vi "Notify Observers (Root).vi"(7 "Type":enum16{"Event", "State"}(ring)=enum."State", 8 "error in (no error)":errorcluster, 10 "Array of State Messages":refnum<class "MSG.lvclass">[](array[class]), 11 "ObserverRegistry in":refnum<class "ObserverRegistry.lvclass">) -> (0 "error out":errorcluster, 3 "ObserverRegistry out":refnum<class "ObserverRegistry.lvclass">)   [LabVIEW 2011, in "Messenging.lvlib" / "ObserverRegistry.lvclass"]
uses:
  ObserverRegistry.lvclass
  Registration Entry.ctl
  Interprocess Messenger/TextVarientMessage/MSG.lvclass
  Interprocess Messenger/SendOnly/Observer.lvclass
  Interprocess Messenger/ErrorMessage/ErrorMessage.lvclass
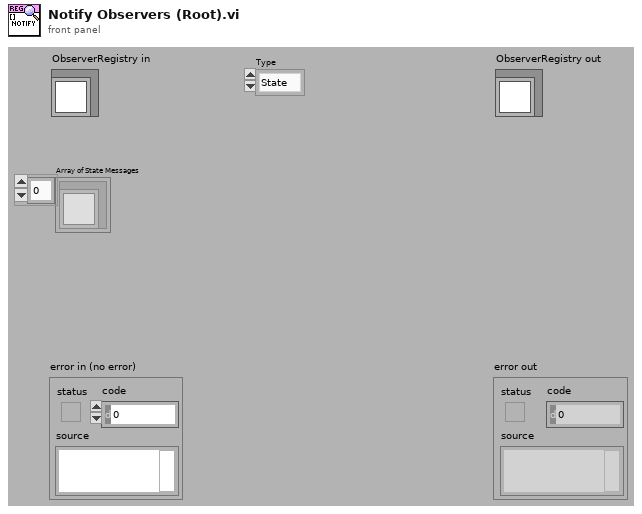
[diagram p1: front panel]
types:
  T1 = typedef "Messenging.lvlib/ObserverRegistry.lvclass/Registration Entry.ctl" = cluster{"Observer":refnum<class "Observer.lvclass">, "Type":enum16{"Event", "State"}, "Latest (State)":refnum<class "MSG.lvclass">}
  T2 = typedef "Messenging.lvlib/ObserverRegistry.lvclass/ObserverRegistryData.ctl" = cluster{"Observer of Errors":refnum<class "Observer.lvclass">, "Observer of All":refnum<class "Observer.lvclass">, "Event Registry":variant}
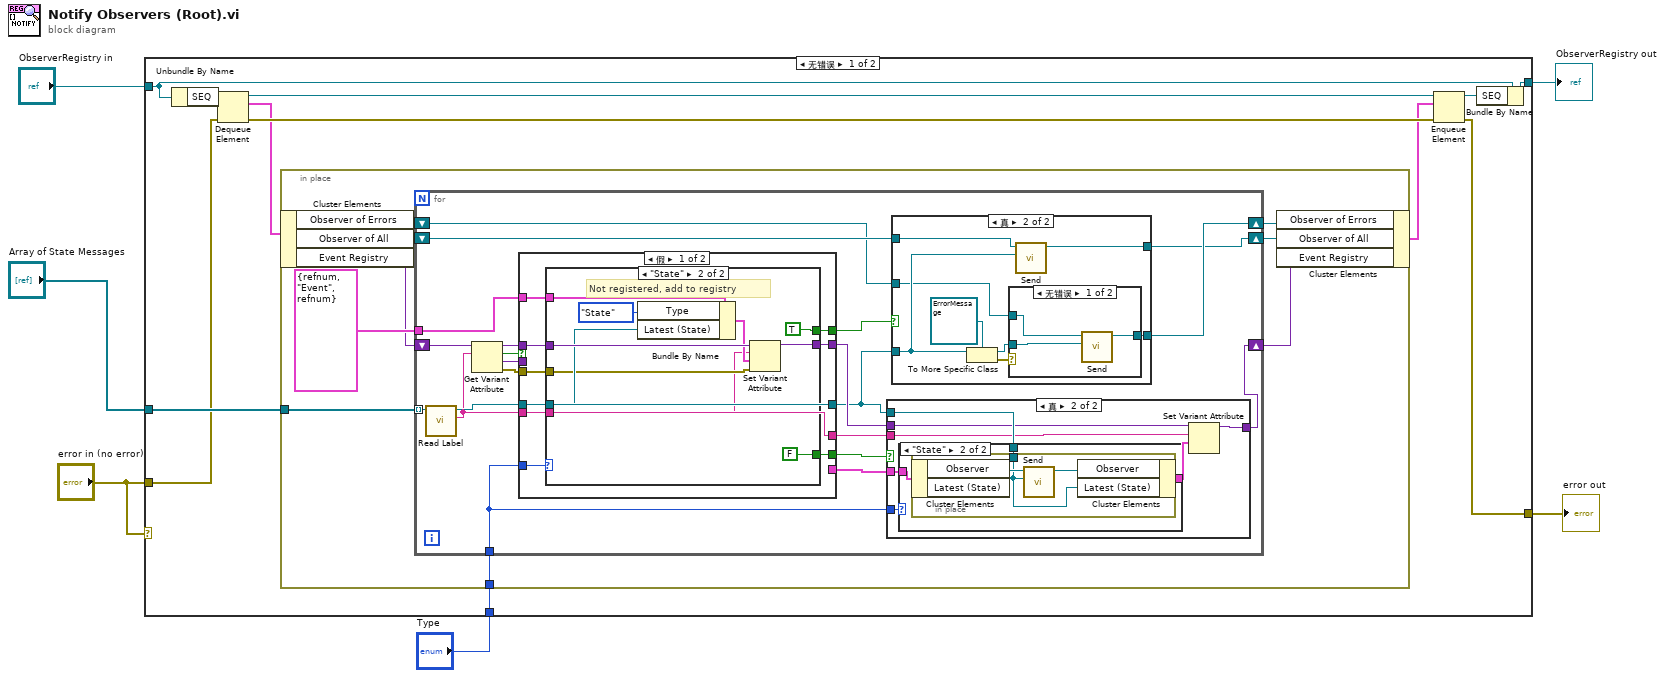
[diagram p0: block diagram]
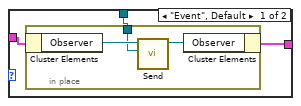
[diagram p3: hidden frame]
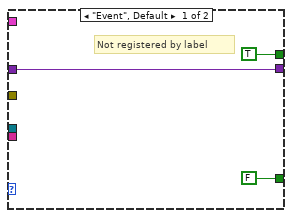
[diagram p6: hidden frame]
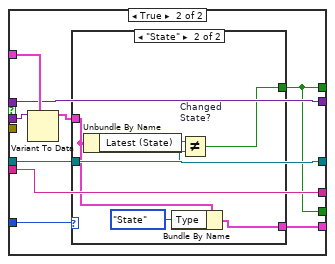
[diagram p7: hidden frame]
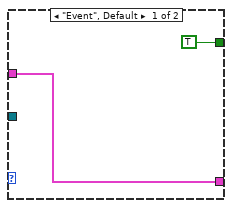
[diagram p8: hidden frame]
diagram:
  n1 = case shown="无错误" "error in (no error)" {
    tunnel: "ObserverRegistry in" -> [w18 w122]
    tunnel: [w17 w122] -> w5
    tunnel: [w16 w123] -> w4
    tunnel: "Array of State Messages" -> [w9 _]
    tunnel: "error in (no error)" -> [w8 w123]
    tunnel: "Type" -> [w7 _]
    frame No Error {
      n2 = Unbundle By Name(w18) -> ("SEQ"=w15:refnum<queue>)
      n3 = Dequeue Element(queue=w15, error in (no error)=w8) -> (queue out=w13:refnum<queue>, element=w11:T2, error out=w12:errorcluster)  [unwired: 2 out]
      n4 = in-place {
        in-place-border: w9 -> [w27]
        in-place-border: w7 -> [w19]
        n5 = in-place-cluster #1(w11) -> ("Observer of Errors"=w23:refnum<class "Observer.lvclass">, "Observer of All"=w24:refnum<class "Observer.lvclass">, "Event Registry"=w25:variant)
        n6 = for {
          tunnel: w27 -> [w48] mode=indexing
          tunnel: T1 {"Observer"=refnum, "Type"=enum."Event", "Latest (State)"=refnum} ("Registration Entry") -> [w44]
          shift-right: [w36] -> w22
          shift-left: w23 -> [w37]
          shift-right: [w35] -> w21
          shift-left: w24 -> [w38]
          shift-right: [w29] -> w20
          shift-left: w25 -> [w39]
          tunnel: w19 -> [w28]
          n7 = call-dynamic "Read Label.vi"("Message"=w48) -> ("Label"=w42:string, "Message"=w45:refnum<class "MSG.lvclass">)  [unwired: 1 in, 8 out]
          n8 = Get Variant Attribute(Variant=w39, name=w42) -> (duplicate Variant=w43:variant, found=w47:bool, value=w46:variant, error out=w40:errorcluster)  [unwired: 2 in]
          n9 = case shown="假" w47 {
            tunnel: w46 -> [_ w113]
            tunnel: w44 -> [w91 w112]
            tunnel: w45 -> [w89 w108]
            tunnel: w43 -> [w90 w111]
            tunnel: w42 -> [w84 w110]
            tunnel: [w89 w108] -> w31
            tunnel: [w88 w105] -> w41
            tunnel: w40 -> [w87 _]
            tunnel: [w86 w111] -> w32
            tunnel: [w85 w105] -> w34
            tunnel: [_ w109] -> w33
            tunnel: [w84 w110] -> w30
            tunnel: w28 -> [w83 w106]
            frame False {
              n10 = case shown="\"State\"" w83 {
                tunnel: w91 -> [_ w104]
                tunnel: w90 -> [w94 w102]
                tunnel: w89 -> [_ w101]
                tunnel: [TRUE TRUE] -> w88
                tunnel: w87 -> [_ w98]
                tunnel: [w94 w97] -> w86
                tunnel: [FALSE FALSE] -> w85
                tunnel: w84 -> [_ w95]
                frame "Event", Default {
                  # "Not registered by label"
                }
                frame "State" {
                  # "Not registered, add to registry"
                  n11 = Bundle By Name(cluster=w104, "Type"=enum16{"Event", "State"}."State", "Latest (State)"=w101) -> (w100:T1)
                  n12 = Set Variant Attribute(Variant=w102, name=w95, value=w100, error in=w98) -> (Variant out=w97:variant)  [unwired: 2 out]
                }
              }
            }
            frame True {
              n13 = Variant To Data(type=w112, Variant=w113) -> (data=w107:T1)  [unwired: 1 in, 1 out]
              n14 = case shown="\"State\"" w106 {
                tunnel: [w114 w121] -> w109
                tunnel: [TRUE w116] -> w105
                tunnel: w108 -> [_ w120]
                tunnel: w107 -> [w114 w118]
                frame "Event", Default {
                }
                frame "State" {
                  n15 = Unbundle By Name(w118) -> ("Latest (State)"=w119:refnum<class "MSG.lvclass">)
                  n16 = Bundle By Name(cluster=w118, "Type"=enum16{"Event", "State"}."State") -> (w121:T1)
                  n17 = Not Equal? "Changed\nState?"(x=w119, y=w120) -> (x != y?=w116:bool)
                }
              }
            }
          }
          n18 = case shown="真" w34 {
            tunnel: w33 -> [_ w56]
            tunnel: w32 -> [w49 w54]
            tunnel: w31 -> [_ w55]
            tunnel: w30 -> [_ w52]
            tunnel: [w49 w51] -> w29
            tunnel: w28 -> [_ w50]
            frame False {
            }
            frame True {
              n19 = case shown="\"State\"" w50 {
                tunnel: w56 -> [w59 w65]
                tunnel: w55 -> [w58 w64]
                tunnel: [w57 w63] -> w53
                frame "Event", Default {
                  n20 = in-place {
                    in-place-border: w58 -> [w60]
                    n21 = in-place-cluster #2(w59) -> ("Observer"=w62:refnum<class "Observer.lvclass">)
                    n22 = call-dynamic "Send.vi"("Message"=w60, "MSR Parent in"=w62) -> ("MSR Parent out"=w61:refnum<class "Observer.lvclass">)  [unwired: 1 in, 8 out]
                    n23 = in-place-cluster #2("Observer"=w61) -> (w57:T1)
                  }
                }
                frame "State" {
                  n24 = in-place {
                    in-place-border: w64 -> [w66]
                    n25 = in-place-cluster #3(w65) -> ("Observer"=w68:refnum<class "Observer.lvclass">)  [unwired: 1 out]
                    n26 = call-dynamic "Send.vi"("Message"=w66, "MSR Parent in"=w68) -> ("MSR Parent out"=w67:refnum<class "Observer.lvclass">)  [unwired: 1 in, 8 out]
                    n27 = in-place-cluster #3("Observer"=w67, "Latest (State)"=w66) -> (w63:T1)
                  }
                }
              }
              n28 = Set Variant Attribute(Variant=w54, name=w52, value=w53) -> (Variant out=w51:variant)  [unwired: 1 in, 2 out]
            }
          }
          n29 = case shown="真" w41 {
            tunnel: w31 -> [_ w75]
            tunnel: w38 -> [w70 w74]
            tunnel: w37 -> [w69 w73]
            tunnel: [w69 w72] -> w36
            tunnel: [w70 w71] -> w35
            frame False {
              # "State not changed --> no notification"
            }
            frame True {
              n30 = To More Specific Class(target class=refnum<class "ErrorMessage.lvclass"> refnum ("Messenging.lvlib:ErrorMessage.lvclass"), reference=w75) -> (specific class reference=w76:refnum<class "ErrorMessage.lvclass">, error out=w77:errorcluster)  [unwired: 1 in]
              n31 = case shown="无错误" w77 {
                tunnel: w73 -> [w80 w82]
                tunnel: w76 -> [w81 _]
                tunnel: [w79 w82] -> w72
                frame No Error {
                  n32 = call-dynamic "Send.vi"("Message"=w81, "MSR Parent in"=w80) -> ("MSR Parent out"=w79:refnum<class "Observer.lvclass">)  [unwired: 1 in, 8 out]
                }
                frame Error {
                }
              }
              n33 = call-dynamic "Send.vi"("Message"=w75, "MSR Parent in"=w74) -> ("MSR Parent out"=w71:refnum<class "Observer.lvclass">)  [unwired: 1 in, 8 out]
            }
          }
        }
        n34 = in-place-cluster #1("Observer of Errors"=w22, "Observer of All"=w21, "Event Registry"=w20) -> (w10:T2)
      }
      n35 = Enqueue Element(queue=w13, element=w10, error in (no error)=w12) -> (queue out=w14:refnum<queue>, error out=w16:errorcluster)  [unwired: 2 out]
      n36 = Bundle By Name(cluster=w18, "SEQ"=w14) -> (w17:refnum<class "ObserverRegistry.lvclass">)
    }
    frame Error {
    }
  }
  "error out" <- w4
  "ObserverRegistry out" <- w5
